vi "5_1_graph.vi"() -> ()   [LabVIEW 2018]
uses:
  <vilib>/ptbypt/NI_PtbyPt.lvlib
panel:
  out "XY Graph 2":cluster{"Y":dbl[], "Y":dbl[]}[](graph) caption="XY图"
  out "XY Graph":cluster{"Y":dbl[], "Y":dbl[]}[](graph) caption="XY图"
  in  "噪声方差":dbl[](array[numeric])
  out "先验概率P(H1)":dbl
  in  "先验概率P(H0)":dbl=0.46
  in  "样本数":u64=1000000
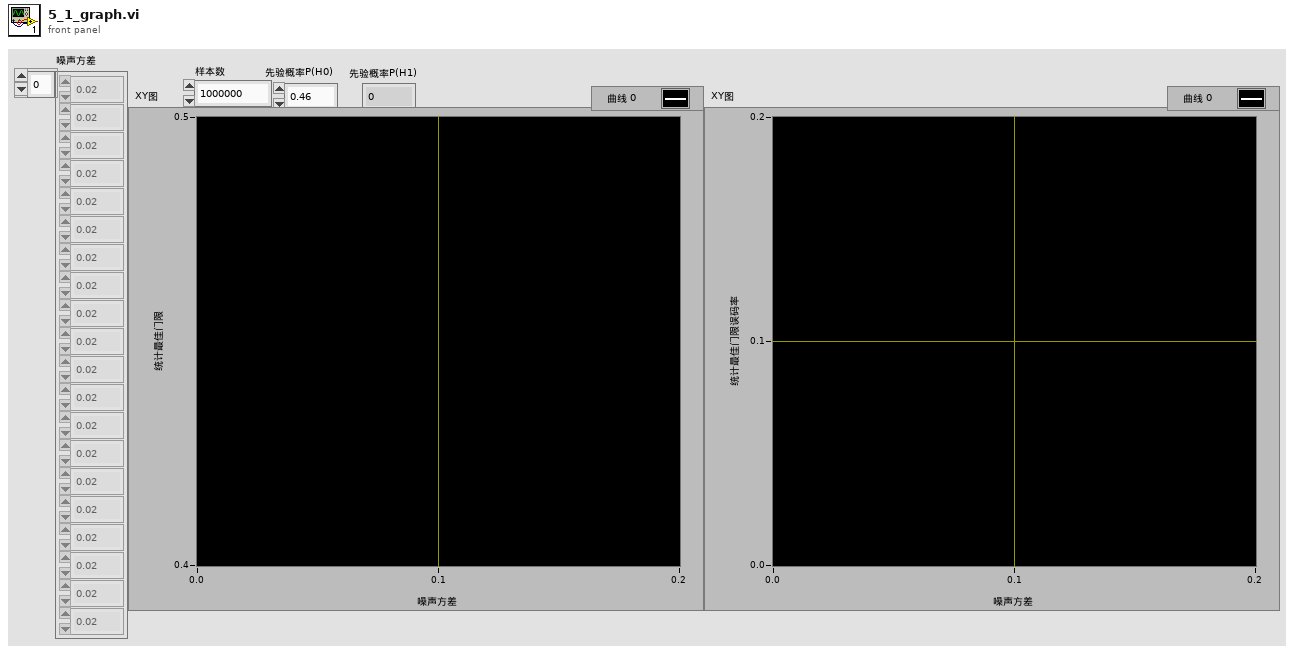
[diagram p1: front panel]
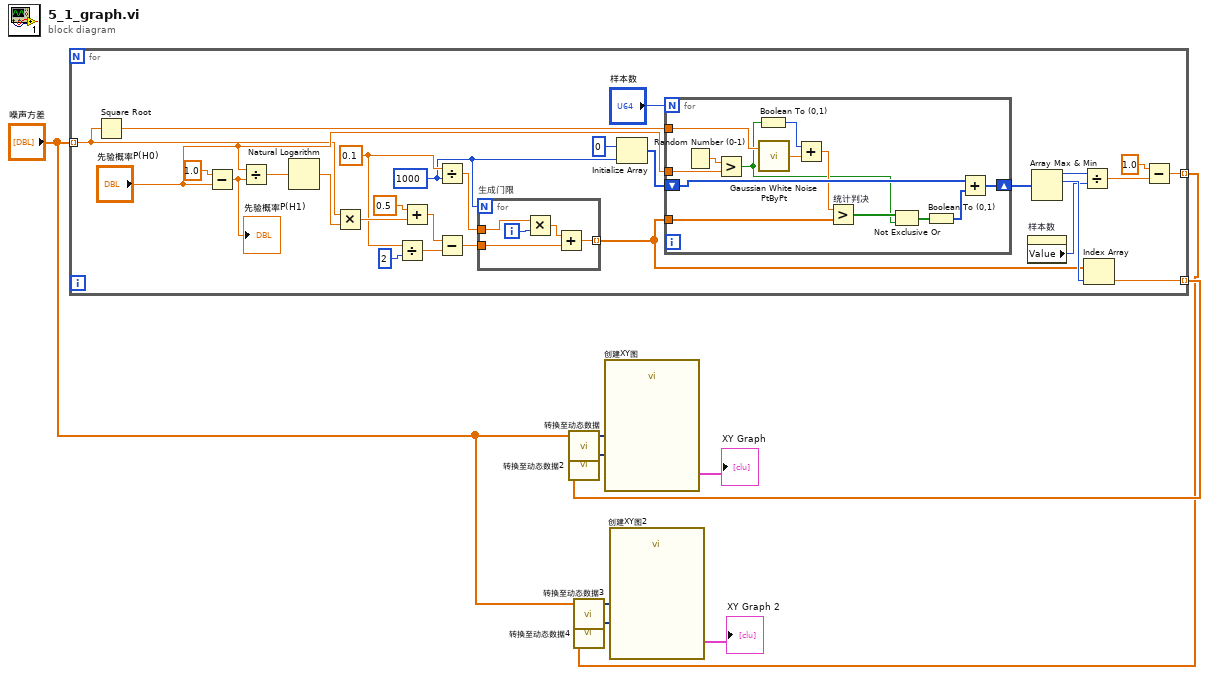
[diagram p0: block diagram]
diagram:
  n1 = for {
    tunnel: "噪声方差" -> [w12] mode=indexing
    tunnel: [w11] -> w2 mode=indexing
    tunnel: [w10] -> w6 mode=indexing
    w27 = 0.1 ("x")
    w20 = u64 1000
    n2 = Square Root(x=w12) -> (sqrt(x)=w15:dbl)
    n3 = Subtract(x=1.0, y="先验概率P(H0)") -> (x-y=w19:dbl)
    "先验概率P(H1)" <- w19
    n4 = Divide(x="先验概率P(H0)", y=w19) -> (x/y=w35:dbl)
    n5 = Natural Logarithm(1:w35) -> (0:w34:dbl)
    n6 = Multiply(x=w12, y=w34) -> (x*y=w33:dbl)
    n7 = Divide(x=w27, y=u64 2) -> (x/y=w28:dbl)
    n8 = Add(x=0.5, y=w33) -> (x+y=w17:dbl)
    n9 = Divide(x=w27, y=w20) -> (x/y=w30:dbl)
    n10 = Subtract(x=w17, y=w28) -> (x-y=w29:dbl)
    n11 = for "生成门限" {
      N: w20 -> [_]
      tunnel: w30 -> [w41]
      tunnel: [w39] -> w21 mode=indexing
      tunnel: w29 -> [w38]
      i -> [w42]
      n12 = Multiply(x=w41, y=w42) -> (x*y=w40:dbl)
      n13 = Add(x=w40, y=w38) -> (x+y=w39:dbl)
    }
    n14 = Initialize Array(u64 0 ("元素"), w20) -> (w24:u64[])
    n15 = for {
      N: "样本数" -> [_]
      tunnel: w15 -> [w55]
      tunnel: "先验概率P(H0)" -> [w52]
      tunnel: w21 -> [w51]
      shift-right: [w48] -> w23
      shift-left: w24 -> [w49]
      n16 = Random Number (0-1)() -> (number: 0 to 1=w53:dbl)
      n17 = Greater?(x=w53, y=w52) -> (0:w43:bool)
      n18 = Boolean To (0,1)(Boolean=w43) -> (0, 1=w46:i16)
      n19 = call <vilib>:"Gaussian White Noise PtByPt.vi"("standard deviation"=w55) -> ("Gaussian white noise"=w54:dbl)  [unwired: 2 in]
      n20 = Add(x=w46, y=w54) -> (x+y=w44:dbl)
      n21 = Greater? "统计判决"(x=w44, y=w51) -> (0:w47:bool[])
      n22 = Not Exclusive Or(1:w43, 2:w47) -> (0:w45:bool[])
      n23 = Boolean To (0,1)(Boolean=w45) -> (0, 1=w50:i16[])
      n24 = Add(x=w49, y=w50) -> (x+y=w48:u64[])
    }
    n25 = property on="样本数" class="DigNum (严格)"() -> ("Value"=w18:u64)  [unwired: 2 in, 2 out]
    n26 = Array Max & Min(array=w23) -> (max value=w16:u64, max index (indices)=w22:i32)  [unwired: 2 out]
    n27 = Divide(x=w16, y=w18) -> (x/y=w14:dbl)
    n28 = Index Array(array=w21, index=w22) -> (element=w10:dbl)
    n29 = Subtract(x=1.0, y=w14) -> (x-y=w11:dbl)
  }
  n30 = call "转换至动态数据"("Array"="噪声方差") -> ("Dynamic Data Type"=w7:dynamicdata)  [unwired: 3 in]
  n31 = call "转换至动态数据2"("Array"=w6) -> ("Dynamic Data Type"=w5:dynamicdata)  [unwired: 3 in]
  n32 = call "转换至动态数据3"("Array"="噪声方差") -> ("Dynamic Data Type"=w3:dynamicdata)  [unwired: 3 in]
  n33 = call "转换至动态数据4"("Array"=w2) -> ("Dynamic Data Type"=w1:dynamicdata)  [unwired: 3 in]
  n34 = call "创建XY图"("Y Input"=w5, "X Input"=w7) -> ("XY Graph"=→"XY Graph":cluster{"X":dbl[], "Y":dbl[]}[])  [unwired: 8 in, 1 out]
  n35 = call "创建XY图2"("Y Input"=w1, "X Input"=w3) -> ("XY Graph"=→"XY Graph 2":cluster{"X":dbl[], "Y":dbl[]}[])  [unwired: 8 in, 1 out]
